vi "DAQ.Write AO.vi"(8 "error in (no error)":errorcluster, 10 "AO []":waveform(dbl)[](array[waveform]), 11 "Instrument.DAQ in":refnum<class "Instrument.DAQ.lvclass">) -> (0 "error out":errorcluster, 2 "AO out []":waveform(dbl)[](array[waveform]), 3 "Instrument.DAQ out":refnum<class "Instrument.DAQ.lvclass">, 4 "AO time (ms)":u32=53)   [LabVIEW 2019, in "Instrument.Lockin.lvlib" / "Instrument.DAQ.lvclass"]
uses:
  Instrument.DAQ.lvclass
  Instrument.DAQ.lvclass/Instrument.DAQ.ctl
  <vilib>/DAQmx/write.llb/DAQmx Write (Analog 1D Wfm NChan NSamp).vi
  <vilib>/Waveform/WDTOps.llb/WDT Append Waveforms DBL.vi
  <vilib>/DAQmx/miscellaneous.llb/DAQmx Fill In Error Info.vi
panel:
  out "AO (previous)":waveform(dbl)[](array[waveform])
  out "Waveform Graph":waveform(dbl)[](graph)
  out "P Check":bool[](array[boolean])
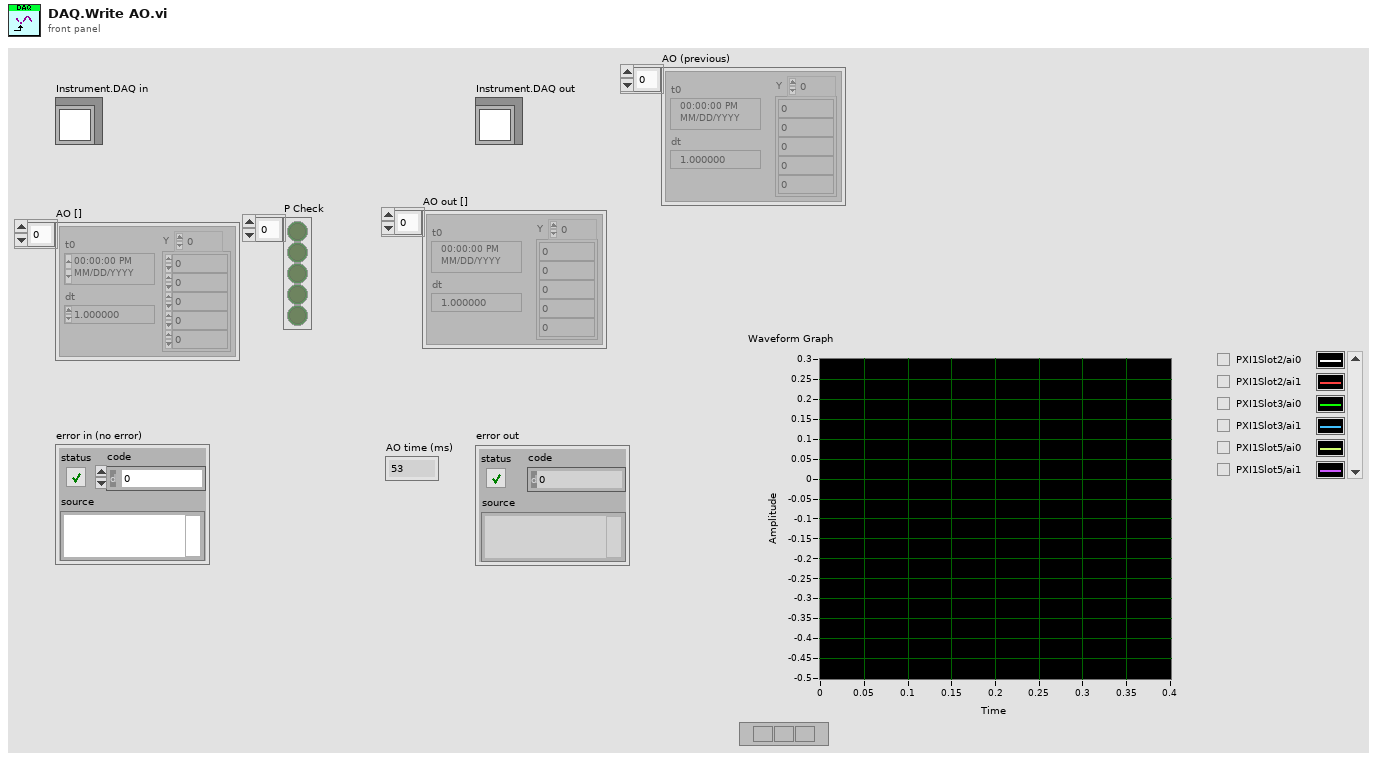
[diagram p1: front panel]
types:
  T1 = enum16{"static", "dynamic", "dynamic asynchronous"}
  T2 = typedef "Instrument.Lockin.lvlib/Instrument.DAQ.lvclass/DAQ.Type--enum.ctl" = enum16{"None", "USB-4431", "PXI-446x"}
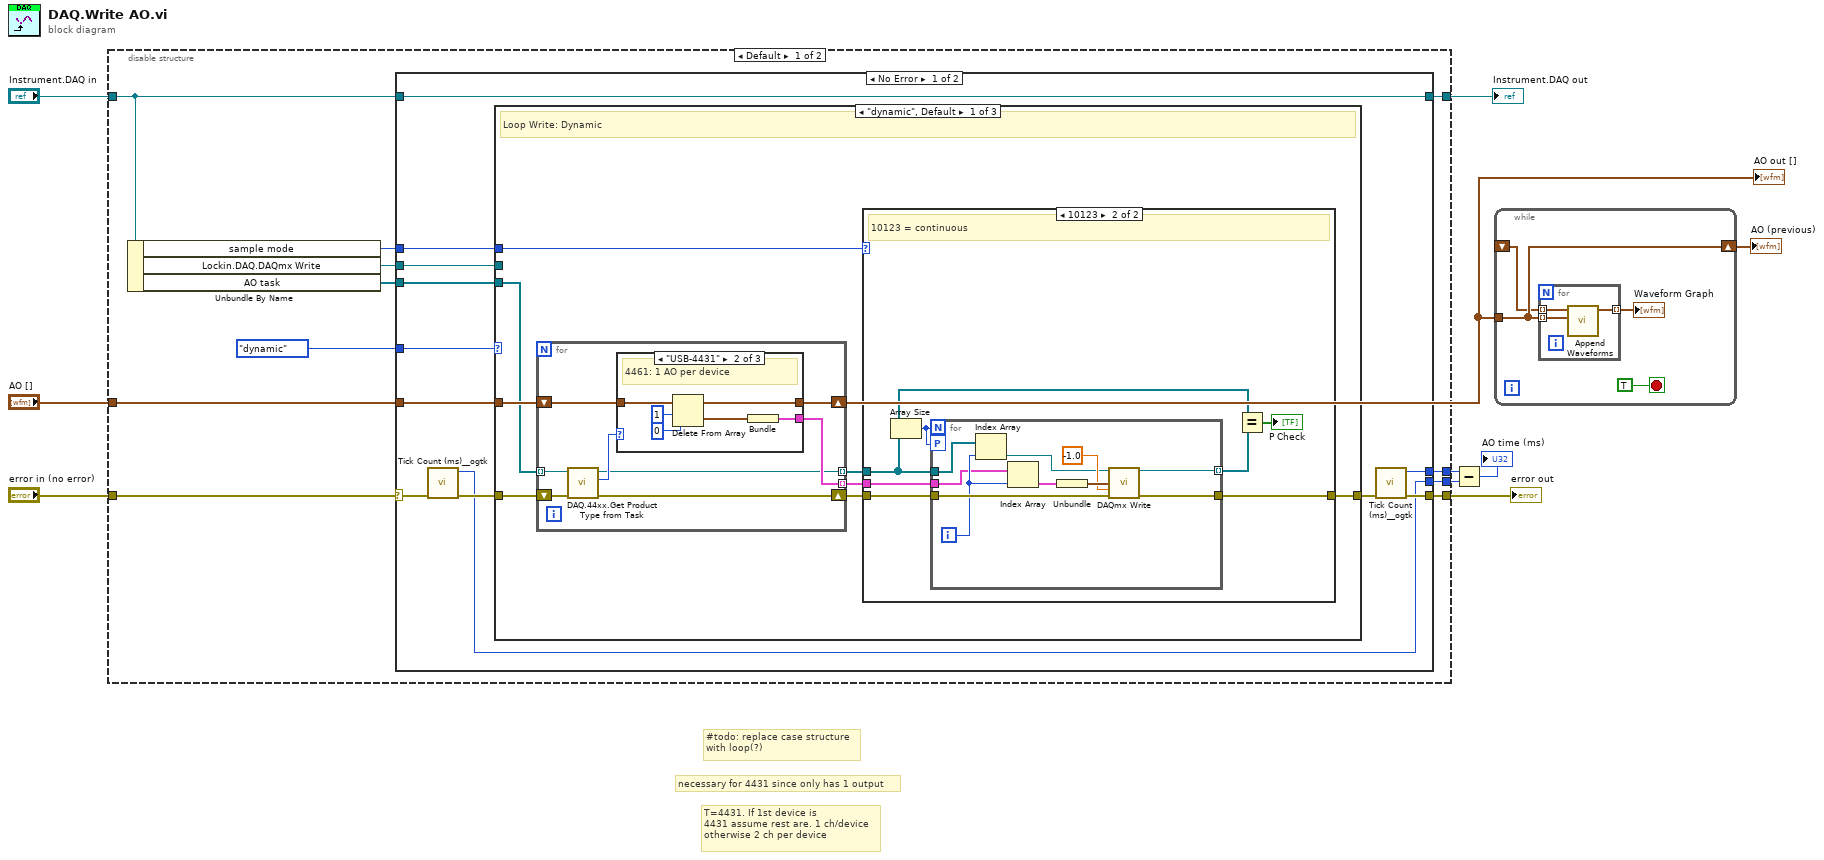
[diagram p0: block diagram]
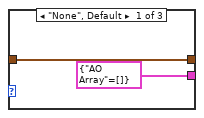
[diagram p2: hidden frame]
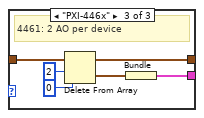
[diagram p3: hidden frame]
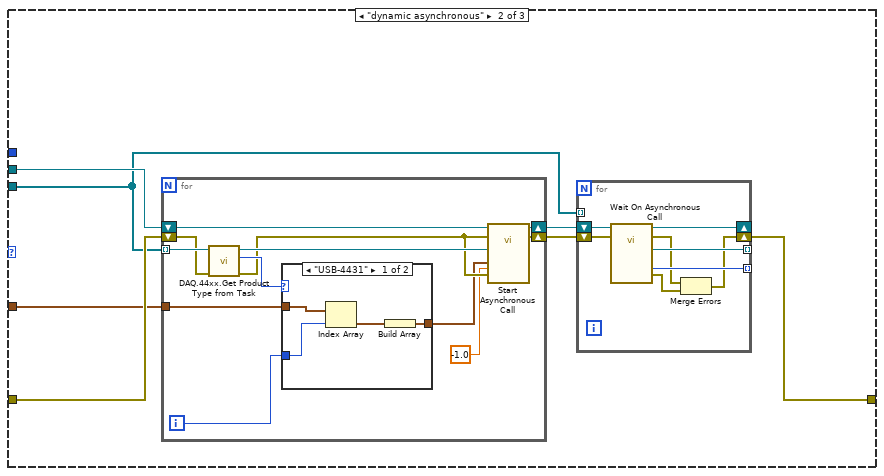
[diagram p5: hidden frame]
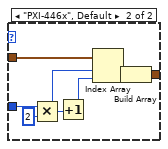
[diagram p6: hidden frame]
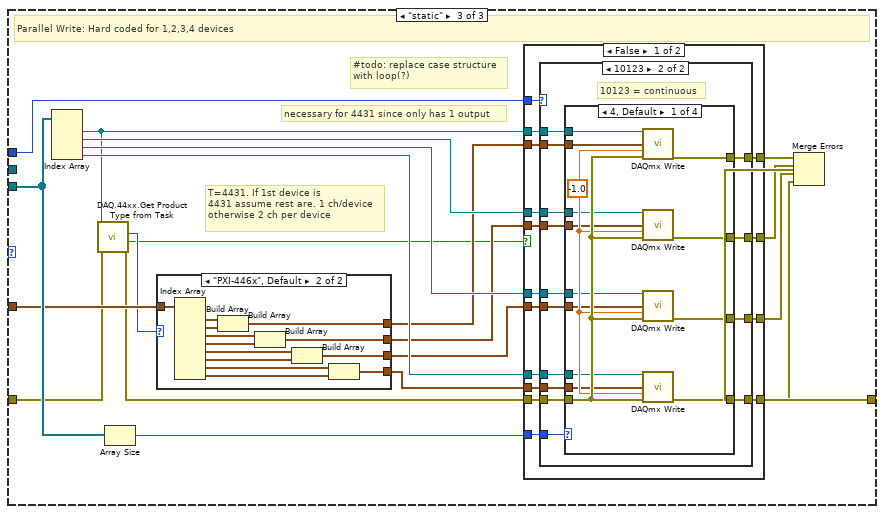
[diagram p7: hidden frame]
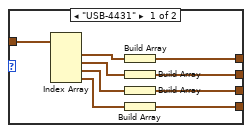
[diagram p8: hidden frame]
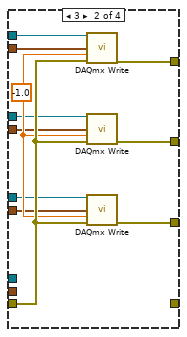
[diagram p10: hidden frame]
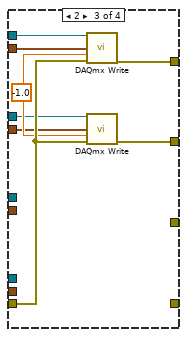
[diagram p11: hidden frame]
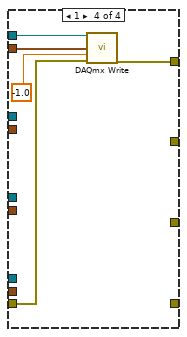
[diagram p12: hidden frame]
diagram:
  # "#todo: replace case structure\nwith loop(?)"
  # "T=4431. If 1st device is \n4431 assume rest are. 1 ch/device\notherwise 2 ch per device"
  # "necessary for 4431 since only has 1 output"
  n1 = disable-structure shown="Default" {
    disable-tunnel: [w20 w235] -> w7
    disable-tunnel: "Instrument.DAQ in" -> [w18 w234]
    disable-tunnel: "AO []" -> [w19 _]
    disable-tunnel: "error in (no error)" -> [w13 w235]
    disable-tunnel: [w17 w234] -> w6
    disable-tunnel: [w16 _] -> w9
    disable-tunnel: [w15 _] -> w4
    frame condition #0 (active) {
      n2 = Unbundle By Name(w18) -> ("sample mode"=w10:i32, "Lockin.DAQ.DAQmx Write"=w12:refnum<vi>, "AO task"=w14:refnum<k21>[])
      n3 = case shown="No Error" w13 {
        selector: w13 -> [w26 w232]
        tunnel: [w29 w232] -> w20
        tunnel: w19 -> [w31 _]
        tunnel: w14 -> [w32 _]
        tunnel: w18 -> [w27 w233]
        tunnel: [w27 w233] -> w17
        tunnel: [w28 _] -> w16
        tunnel: [w23 _] -> w15
        tunnel: w12 -> [w24 _]
        tunnel: T1."dynamic" ("Enum") -> [w22 _]
        tunnel: w10 -> [w21 _]
        frame No Error {
          n4 = call <userlib>:"Tick Count (ms)__ogtk.vi"("error in (no error)"=w26) -> ("error out"=w25:errorcluster, "millisecond timer value"=w23:u32)  [unwired: 9 in]
          n5 = case shown="\"dynamic\", Default" w22 {
            tunnel: w32 -> [w34 w81 w140]
            tunnel: w31 -> [w38 w83 w139]
            tunnel: [w37 w82 w138] -> w30
            tunnel: w25 -> [w40 w85 w123]
            tunnel: w24 -> [_ w84 _]
            tunnel: w21 -> [w33 _ w120]
            frame "dynamic", Default {
              # "Loop Write: Dynamic"
              n6 = for {
                tunnel: [w44] -> w36 mode=indexing
                shift-right: [w47] -> w39
                shift-left: w40 -> [w48]
                tunnel: w34 -> [w43] mode=indexing
                shift-right: [w42] -> _
                shift-left: w38 -> [w46]
                tunnel: [w41] -> w35 mode=indexing
                n7 = call "DAQ.44xx.Get Product Type from Task.vi"("error in (no error)"=w48, "Refnum in"=w43) -> ("error out"=w47:errorcluster, "DAQ Type"=w45:T2, "Refnum out"=w41:refnum<k21>)  [unwired: 6 in, 1 out]
                n8 = case shown="\"USB-4431\"" w45 {
                  tunnel: w46 -> [w50 w56 w62]
                  tunnel: [w50 w55 w61] -> w42
                  tunnel: [cluster{"AO Array":waveform(dbl)[]} {"AO Array"=[]} w53 w58] -> w44
                  frame "None", Default {
                  }
                  frame "USB-4431" {
                    # "4461: 1 AO per device"
                    n9 = Delete From Array(array=w56, length=1, index=0) -> (deleted portion=w52:waveform(dbl)[], array with subset deleted=w55:waveform(dbl)[])
                    n10 = Bundle("AO []"=w52) -> (w53:cluster{"AO []":waveform(dbl)[]})  [unwired: 1 in]
                  }
                  frame "PXI-446x" {
                    # "4461: 2 AO per device"
                    n11 = Delete From Array(array=w62, length=2, index=0) -> (deleted portion=w59:waveform(dbl)[], array with subset deleted=w61:waveform(dbl)[])
                    n12 = Bundle("AO []"=w59) -> (w58:cluster{"AO []":waveform(dbl)[]})  [unwired: 1 in]
                  }
                }
              }
              n13 = case shown="10123" w33 {
                tunnel: [w63 w68] -> w37
                tunnel: w35 -> [_ w67]
                tunnel: w36 -> [_ w70]
                tunnel: w39 -> [w63 w69]
                frame 10178, Default {
                  # "10178 = finite sample mode (IV\nmode). Do not try to write\nmore samples to the buffer"
                }
                frame 10123 {
                  # "10123 = continuous"
                  n14 = Array Size(array=w67) -> (size(s)=w65:i32)
                  n15 = for {
                    N: w65 -> [_]
                    tunnel: w67 -> [w73]
                    tunnel: w70 -> [w74]
                    tunnel: w69 -> [w80]
                    tunnel: [w71] -> w68
                    workers-P: w65 -> [_]
                    tunnel: [w72] -> w64 mode=indexing
                    i -> [w75]
                    n16 = Index Array(array=w73, index=w75) -> (element=w76:refnum<k21>)
                    n17 = Index Array(array=w74, index=w75) -> (element=w77:cluster{"AO []":waveform(dbl)[]})
                    n18 = Unbundle(w77) -> ("AO []"=w79:waveform(dbl)[])
                    n19 = call-poly <vilib>:"DAQmx Write.vi"("task/channels in"=w76, "data"=w79, "timeout"=-1.0, "error in"=w80) -> ("task out"=w72:refnum<k21>, "error out"=w71:errorcluster)  [unwired: 9 in, 1 out]
                  }
                  n20 = Equal?(x=w67, y=w64) -> (x = y?=→"P Check":bool[])
                }
              }
            }
            frame "dynamic asynchronous" {
              n21 = for {
                shift-right: [w99] -> w86
                shift-left: w85 -> [w93]
                shift-right: [w98] -> w87
                shift-left: w84 -> [w97]
                tunnel: w81 -> [w95] mode=indexing
                tunnel: w83 -> [w91]
                i -> [w90]
                n22 = call "DAQ.44xx.Get Product Type from Task.vi"("error in (no error)"=w93, "Refnum in"=w95) -> ("error out"=w92:errorcluster, "DAQ Type"=w96:T2, "Refnum out"=w94:refnum<k21>)  [unwired: 6 in, 1 out]
                n23 = case shown="\"USB-4431\"" w96 {
                  tunnel: [w102 w109] -> w89
                  tunnel: w91 -> [w101 w108]
                  tunnel: w90 -> [w100 w106]
                  frame "USB-4431" {
                    n24 = Index Array(array=w101, index=w100) -> (element=w103:waveform(dbl))
                    n25 = Build Array(w103) -> (w102:waveform(dbl)[])
                  }
                  frame "PXI-446x", Default {
                    n26 = Multiply(x=w106, y=2) -> (x*y=w105:i32)
                    n27 = Increment(x=w105) -> (x+1=w104:i32)
                    n28 = Index Array(array=w108, index #1=w105, index #2=w104) -> (element #1=w110:waveform(dbl), element #2=w111:waveform(dbl))
                    n29 = Build Array(w110, w111) -> (w109:waveform(dbl)[])
                  }
                }
                n30 = call-by-ref "Start Asynchronous Call"(reference=w97, error in=w92, "Refnum in"=w94, "data"=w89, "timeout"=-1.0, 11:"error in (no error)"=w92) -> (reference out=w98:refnum<vi>, error out=w99:errorcluster)  [unwired: 8 in, 4 out]
              }
              n31 = for {
                shift-right: [w112] -> w82
                shift-left: w86 -> [w118]
                shift-right: [w117] -> _
                shift-left: w87 -> [w119]
                tunnel: [w116] -> _ mode=indexing
                tunnel: [w115] -> _ mode=indexing
                tunnel: w81 -> [_] mode=indexing
                n32 = call-by-ref "Wait On Asynchronous Call"(reference=w119, error in=w118) -> (reference out=w117:refnum<vi>, error out=w113:errorcluster, "Refnum out"=w116:refnum<k21>, "number of samples written per channel"=w115:u32, 15:"error out"=w114:errorcluster)  [unwired: 12 in, 1 out]
                n33 = Merge Errors(w113, w114) -> (w112:errorcluster)
              }
            }
            frame "static" {
              # "#todo: replace case structure\nwith loop(?)"
              # "T=4431. If 1st device is \n4431 assume rest are. 1 ch/device\notherwise 2 ch per device"
              # "necessary for 4431 since only has 1 output"
              # "Parallel Write: Hard coded for 1,2,3,4 devices"
              n34 = Index Array(array=w140) -> (element #1=w133:refnum<k21>, element #2=w137:refnum<k21>, element #3=w136:refnum<k21>, element #4=w135:refnum<k21>)  [unwired: 4 in]
              n35 = call "DAQ.44xx.Get Product Type from Task.vi"("error in (no error)"=w123, "Refnum in"=w133) -> ("error out"=w122:errorcluster, "DevIsSimulated"=w124:bool, "DAQ Type"=w129:T2)  [unwired: 6 in, 1 out]
              n36 = Array Size(array=w140) -> (size(s)=w134:i32)
              n37 = case shown="\"PXI-446x\", Default" w129 {
                tunnel: [w149 w155] -> w131
                tunnel: [w148 w154] -> w132
                tunnel: [w147 w153] -> w121
                tunnel: [w145 w151] -> w130
                tunnel: w139 -> [w144 w150]
                frame "USB-4431" {
                  n38 = Index Array(array=w144) -> (element #1=w146:waveform(dbl), element #2=w143:waveform(dbl), element #3=w142:waveform(dbl), element #4=w141:waveform(dbl))  [unwired: 4 in]
                  n39 = Build Array(w146) -> (w145:waveform(dbl)[])
                  n40 = Build Array(w143) -> (w149:waveform(dbl)[])
                  n41 = Build Array(w142) -> (w148:waveform(dbl)[])
                  n42 = Build Array(w141) -> (w147:waveform(dbl)[])
                }
                frame "PXI-446x", Default {
                  n43 = Index Array(array=w150) -> (element #1=w152:waveform(dbl), element #2=w162:waveform(dbl), element #3=w161:waveform(dbl), element #4=w160:waveform(dbl), element #5=w159:waveform(dbl), element #6=w158:waveform(dbl), element #7=w157:waveform(dbl), element #8=w156:waveform(dbl))  [unwired: 8 in]
                  n44 = Build Array(w152, w162) -> (w151:waveform(dbl)[])
                  n45 = Build Array(w161, w160) -> (w155:waveform(dbl)[])
                  n46 = Build Array(w159, w158) -> (w154:waveform(dbl)[])
                  n47 = Build Array(w157, w156) -> (w153:waveform(dbl)[])
                }
              }
              n48 = case shown="False" w124 {
                tunnel: w137 -> [w177 _]
                tunnel: w136 -> [w176 _]
                tunnel: w135 -> [w175 _]
                tunnel: w134 -> [w174 _]
                tunnel: w133 -> [w173 _]
                tunnel: w121 -> [w172 _]
                tunnel: w132 -> [w171 _]
                tunnel: w131 -> [w170 _]
                tunnel: w130 -> [w169 _]
                tunnel: w122 -> [w168 w231]
                tunnel: [w167 _] -> w128
                tunnel: [w166 _] -> w127
                tunnel: [w165 w231] -> w126
                tunnel: [w163 _] -> w125
                tunnel: w120 -> [w164 _]
                frame False {
                  n49 = case shown="10123" w164 {
                    tunnel: w177 -> [_ w192]
                    tunnel: w176 -> [_ w191]
                    tunnel: w175 -> [_ w190]
                    tunnel: [w178 w189] -> w165
                    tunnel: [_ w188] -> w166
                    tunnel: [_ w187] -> w167
                    tunnel: [_ w186] -> w163
                    tunnel: w174 -> [_ w185]
                    tunnel: w173 -> [_ w184]
                    tunnel: w172 -> [_ w183]
                    tunnel: w171 -> [_ w182]
                    tunnel: w170 -> [_ w181]
                    tunnel: w169 -> [_ w180]
                    tunnel: w168 -> [w178 w179]
                    frame 10178, Default {
                      # "10178 = finite sample mode (IV\nmode). Do not try to write\nmore samples to the buffer"
                    }
                    frame 10123 {
                      # "10123 = continuous"
                      n50 = case shown="4, Default" w185 {
                        tunnel: w179 -> [w206 w217 w225 w230]
                        tunnel: w192 -> [w204 w215 w223 _]
                        tunnel: w191 -> [w203 w214 _ _]
                        tunnel: w190 -> [w202 _ _ _]
                        tunnel: w181 -> [w201 w213 w222 _]
                        tunnel: w182 -> [w200 w212 _ _]
                        tunnel: w183 -> [w199 _ _ _]
                        tunnel: [w198 w211 w221 w228] -> w189
                        tunnel: [w197 w210 w220 _] -> w188
                        tunnel: [w196 w209 _ _] -> w187
                        tunnel: [w195 _ _ _] -> w186
                        tunnel: w184 -> [w194 w208 w219 w227]
                        tunnel: w180 -> [w193 w207 w218 w226]
                        frame 4, Default {
                          w205 = -1.0 ("timeout")
                          n51 = call-poly <vilib>:"DAQmx Write.vi"("task/channels in"=w194, "data"=w193, "timeout"=w205, "error in"=w206) -> ("error out"=w198:errorcluster)  [unwired: 9 in, 2 out]
                          n52 = call-poly <vilib>:"DAQmx Write.vi"("task/channels in"=w204, "data"=w201, "timeout"=w205, "error in"=w206) -> ("error out"=w197:errorcluster)  [unwired: 9 in, 2 out]
                          n53 = call-poly <vilib>:"DAQmx Write.vi"("task/channels in"=w203, "data"=w200, "timeout"=w205, "error in"=w206) -> ("error out"=w196:errorcluster)  [unwired: 9 in, 2 out]
                          n54 = call-poly <vilib>:"DAQmx Write.vi"("task/channels in"=w202, "data"=w199, "timeout"=w205, "error in"=w206) -> ("error out"=w195:errorcluster)  [unwired: 9 in, 2 out]
                        }
                        frame 3 {
                          w216 = -1.0 ("timeout")
                          n55 = call-poly <vilib>:"DAQmx Write.vi"("task/channels in"=w208, "data"=w207, "timeout"=w216, "error in"=w217) -> ("error out"=w211:errorcluster)  [unwired: 9 in, 2 out]
                          n56 = call-poly <vilib>:"DAQmx Write.vi"("task/channels in"=w215, "data"=w213, "timeout"=w216, "error in"=w217) -> ("error out"=w210:errorcluster)  [unwired: 9 in, 2 out]
                          n57 = call-poly <vilib>:"DAQmx Write.vi"("task/channels in"=w214, "data"=w212, "timeout"=w216, "error in"=w217) -> ("error out"=w209:errorcluster)  [unwired: 9 in, 2 out]
                        }
                        frame 2 {
                          w224 = -1.0 ("timeout")
                          n58 = call-poly <vilib>:"DAQmx Write.vi"("task/channels in"=w219, "data"=w218, "timeout"=w224, "error in"=w225) -> ("error out"=w221:errorcluster)  [unwired: 9 in, 2 out]
                          n59 = call-poly <vilib>:"DAQmx Write.vi"("task/channels in"=w223, "data"=w222, "timeout"=w224, "error in"=w225) -> ("error out"=w220:errorcluster)  [unwired: 9 in, 2 out]
                        }
                        frame 1 {
                          n60 = call-poly <vilib>:"DAQmx Write.vi"("task/channels in"=w227, "data"=w226, "timeout"=-1.0, "error in"=w230) -> ("error out"=w228:errorcluster)  [unwired: 9 in, 2 out]
                        }
                      }
                    }
                  }
                }
                frame True {
                }
              }
              n61 = Merge Errors(w126, w127, w128, w125) -> (w138:errorcluster)
            }
          }
          n62 = call <userlib>:"Tick Count (ms)__ogtk.vi"("error in (no error)"=w30) -> ("error out"=w29:errorcluster, "millisecond timer value"=w28:u32)  [unwired: 9 in]
        }
        frame Error {
        }
      }
    }
    frame condition #1 {
    }
  }
  "error out" <- w7
  "Instrument.DAQ out" <- w6
  n63 = Subtract(x=w9, y=w4) -> (x-y=→"AO time (ms)":u32)
  n64 = while {
    shift-right: [w237] -> w1
    shift-left: _ -> [w236]
    tunnel: "AO []" -> [w237]
    stop <- TRUE stop-if-true
    n65 = for {
      tunnel: [w242] -> w238 mode=indexing
      tunnel: w236 -> [w241] mode=indexing
      tunnel: w237 -> [w240] mode=indexing
      n66 = call-poly <vilib>:"Append Waveforms.vi"("waveform B"=w240, "waveform A"=w241) -> ("waveform out"=w242:waveform(dbl))  [unwired: 8 in, 1 out]
    }
    "Waveform Graph" <- w238
  }
  "AO (previous)" <- w1
  "AO out []" <- "AO []"
